vi "build_rid.vi"(7 "ext":string="_data.h5", 8 "error in (no error)":errorcluster, 9 "save?":bool, 10 "time stamp":timestamp, 11 "base":path[](array[path])) -> (0 "error out":errorcluster, 2 "run ID":string="20180125_155324", 3 "output":path[](array[path]))   [LabVIEW 2017, in "tools.lvlib"]
uses:
  tools.lvlib
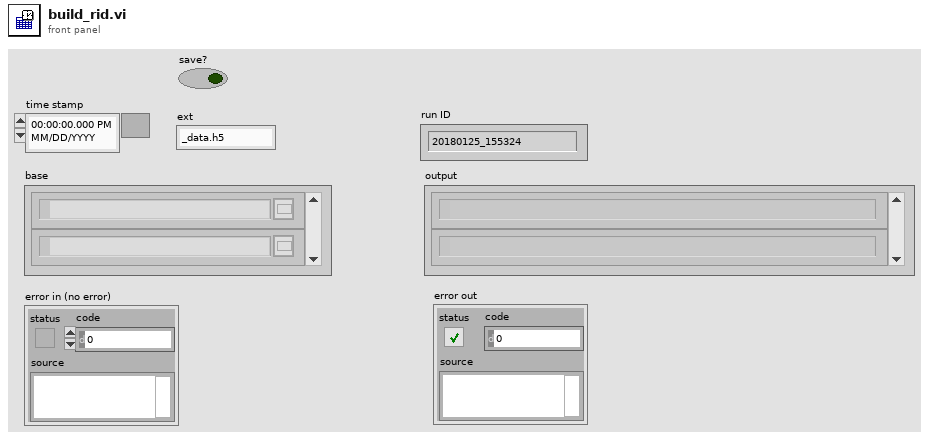
[diagram p1: front panel]
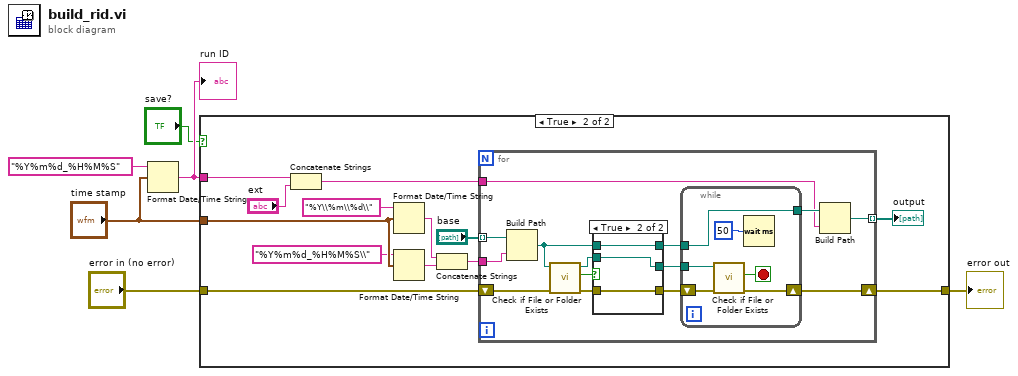
[diagram p0: block diagram]
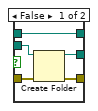
[diagram p3: hidden frame]
diagram:
  n1 = Format Date/Time String(time format string (%c)="%Y%m%d_%H%M%S", seconds (now)="time stamp") -> (date/time string=w4:string)  [unwired: 1 in]
  "run ID" <- w4
  n2 = case shown="True" "save?" {
    tunnel: "time stamp" -> [_ w20]
    tunnel: w4 -> [_ w14]
    tunnel: "error in (no error)" -> [w7 w9]
    tunnel: [w7 w8] -> w1
    frame False {
    }
    frame True {
      n3 = Concatenate Strings(w14, "ext") -> (w11:string)
      n4 = Format Date/Time String(time format string (%c)="%Y\\%m\\%d\\", seconds (now)=w20) -> (date/time string=w16:string)  [unwired: 1 in]
      n5 = Format Date/Time String(time format string (%c)="%Y%m%d_%H%M%S\\", seconds (now)=w20) -> (date/time string=w17:string)  [unwired: 1 in]
      n6 = Concatenate Strings(w16, w17) -> (w12:string)
      n7 = for {
        tunnel: "base" -> [w28] mode=indexing
        tunnel: w12 -> [w27]
        tunnel: w11 -> [w26]
        tunnel: [w25] -> w10 mode=indexing
        shift-right: [w21] -> w8
        shift-left: w9 -> [w23]
        n8 = Build Path(base path=w28, name or relative path=w27) -> (appended path=w30:path)
        n9 = call <vilib>:"Check if File or Folder Exists.vi"("error in (no error)"=w23, "path"=w30) -> ("error out"=w24:errorcluster, "file or folder exists?"=w34:bool, "dup path"=w33:path)  [unwired: 7 in]
        n10 = case shown="True" w34 {
          tunnel: w33 -> [w45 w47]
          tunnel: [w44 w48] -> w31
          tunnel: w30 -> [w44 w48]
          tunnel: [w43 w47] -> w32
          tunnel: w24 -> [w42 w46]
          tunnel: [w41 w46] -> w22
          frame False {
            n11 = Create Folder(path (use dialog)=w45, error in=w42) -> (created path=w43:path, error out=w41:errorcluster)  [unwired: 1 in, 1 out]
          }
          frame True {
          }
        }
        n12 = while {
          tunnel: w32 -> [w39]
          tunnel: [w37] -> w29
          tunnel: w31 -> [w37]
          shift-right: [w35] -> w21
          shift-left: w22 -> [w36]
          stop <- w40 stop-if-true
          n13 = call <vilib>:"Check if File or Folder Exists.vi"("error in (no error)"=w36, "path"=w39) -> ("error out"=w35:errorcluster, "file or folder exists?"=w40:bool)  [unwired: 7 in, 1 out]
          n14 = Wait (ms)(milliseconds to wait=u32 50) -> ()  [unwired: 1 out]
        }
        n15 = Build Path(base path=w29, name or relative path=w26) -> (appended path=w25:path)
      }
      "output" <- w10
    }
  }
  "error out" <- w1
